vi "读取消息.vi"(8 "error in (no error)":errorcluster caption="错误输入（无错误）", 11 "用户操作输入":refnum<class "用户操作.lvclass">) -> (0 "error out":errorcluster caption="错误输出", 2 "操作者框架:消息待入队列":refnum<class "Message Enqueuer.lvclass">, 3 "用户操作输出":refnum<class "用户操作.lvclass">)   [LabVIEW 2020, in "用户操作.lvlib" / "用户操作.lvclass"]
uses:
  <vilib>/ActorFramework/Message Enqueuer/Message Enqueuer.lvclass
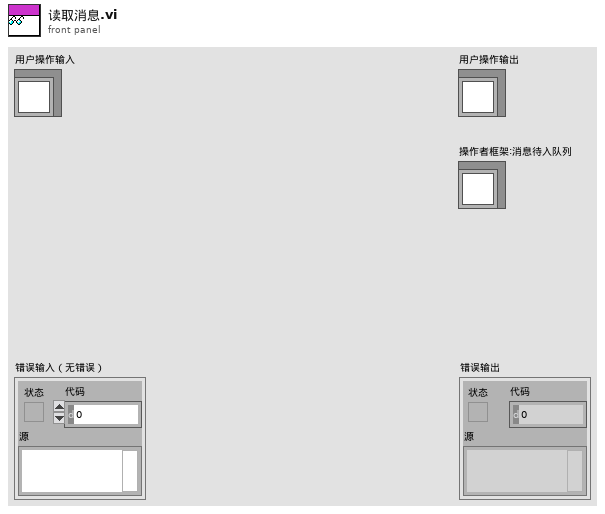
[diagram p1: front panel]
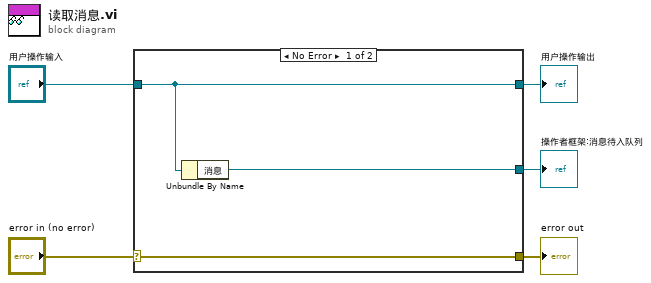
[diagram p0: block diagram]
diagram:
  n1 = case shown="No Error" "error in (no error)" {
    selector: "error in (no error)" -> [w8 w9]
    tunnel: [w8 w9] -> w4
    tunnel: [w7 w10] -> w2
    tunnel: "用户操作输入" -> [w7 w10]
    tunnel: [w6 _] -> w1
    frame No Error {
      n2 = Unbundle By Name(w7) -> ("消息"=w6:refnum<class "Message Enqueuer.lvclass">)
    }
    frame Error {
    }
  }
  "error out" <- w4
  "用户操作输出" <- w2
  "操作者框架:消息待入队列" <- w1
